vi "Register Callbacks.vi"(8 "error in (no error)":errorcluster, 11 "System Definition Tree":T1) -> (0 "error out":errorcluster, 2 "Callbacks":T2, 3 "System Definition Tree dup":T1)   [LabVIEW 2020, in "NI_VS UI System Tree.lvlib"]
uses:
  <vilib>/NI VeriStand/UI Controls/System Definition Tree/NI_VS UI System Tree.lvlib
  <vilib>/NI VeriStand/UI Controls/System Definition Tree/System Definition Tree Ref.ctl
  NationalInstruments.VeriStand.SystemStorageUI
  <vilib>/NI VeriStand/UI Controls/System Definition Tree/Callback Type.ctl
  <vilib>/NI VeriStand/UI Controls/System Definition Tree/Net Event Data Ref.ctl
  <vilib>/NI VeriStand/UI Controls/System Definition Tree/Net Event Data.ctl
  <vilib>/NI VeriStand/UI Controls/System Definition Tree/Net Event.ctl
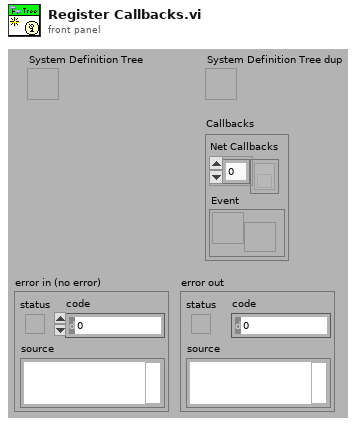
[diagram p1: front panel]
types:
  T1 = typedef "NI_VS UI System Tree.lvlib/System Definition Tree Ref.ctl" = refnum<k24>
  T2 = typedef "NI_VS UI System Tree.lvlib/Callback Type.ctl" = cluster{"Net Callbacks":refnum<k27>[], "Event":T3}
  T3 = typedef "NI_VS UI System Tree.lvlib/Net Event Data Ref.ctl" = refnum<user-event>
  T4 = typedef "NI_VS UI System Tree.lvlib/Net Event Data.ctl" = cluster{"Type":T5, "Data":variant}
  T5 = typedef "NI_VS UI System Tree.lvlib/Net Event.ctl" = enum16{"SelectedItem", "DblClick"}
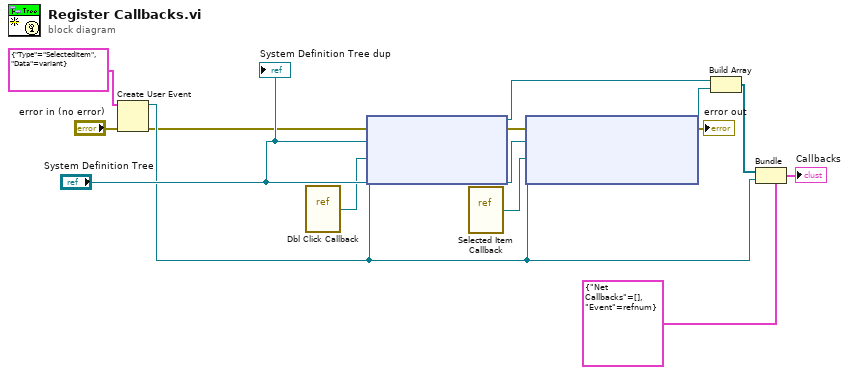
[diagram p0: block diagram]
diagram:
  n1 = Create User Event(user event datatype=T4 {"Type"=enum."SelectedItem", "Data"=variant} ("Net Event Data"), error in="error in (no error)") -> (user event=w4:refnum<user-event>, error out=w1:errorcluster)
  n2 = vi-ref <vilib>:"Dbl Click Callback.vi"() -> ("vi reference"=w11:refnum<vi>)
  n3 = node(w1, "System Definition Tree", w11, w4) -> (w12:refnum<k27>, w10:errorcluster)  [unwired: 1 in]
  n4 = vi-ref <vilib>:"Selected Item Callback.vi"() -> ("vi reference"=w9:refnum<vi>)
  n5 = node(w10, "System Definition Tree", w9, w4) -> (w13:refnum<k27>, →"error out":errorcluster)  [unwired: 1 in]
  n6 = Build Array(w12, w13) -> (w5:refnum<k27>[])
  n7 = Bundle(cluster=T2 {"Net Callbacks"=[], "Event"=refnum} ("Callback"), "Net Callbacks"=w5, "Event"=w4) -> (→"Callbacks":T2)
  "System Definition Tree dup" <- "System Definition Tree"
